vi "Ping_mean.vi"() -> ()   [LabVIEW 2018]
uses:
  <vilib>/Analysis/NI_AALBase.lvlib
panel:
  out "Distance (m)":dbl
  out "median":dbl format="%0.2f"
  in  "Count Integer":i32
  out "Last 10 (2)":dbl[](array[numeric]) format="%.3f"
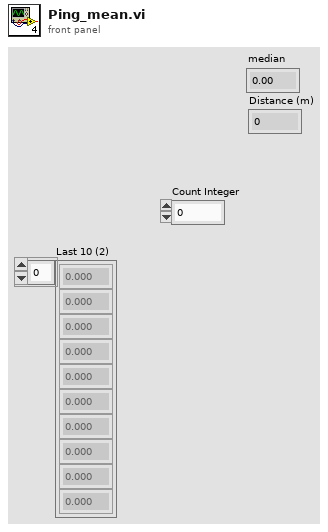
[diagram p1: front panel]
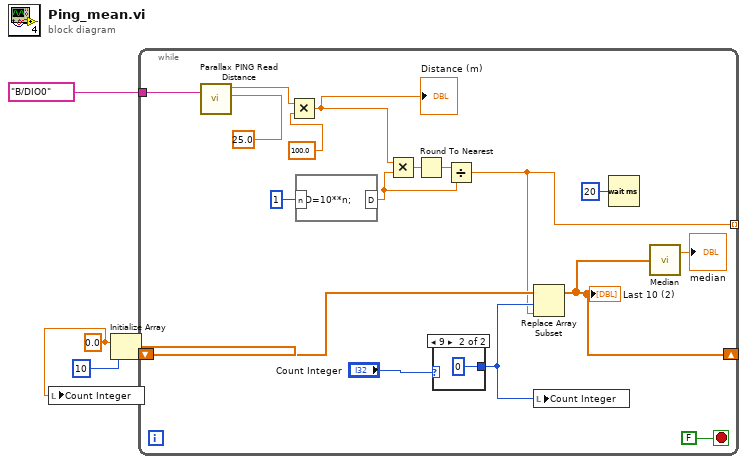
[diagram p0: block diagram]
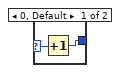
[diagram p2: hidden frame]
diagram:
  w2 = 0.0 ("element")
  n1 = local write "Count Integer"(w2) -> ()
  n2 = Initialize Array(w2, 10 ("dimension size")) -> (w3:dbl[])
  n3 = while {
    shift-right: [w16] -> _
    shift-left: w3 -> [w21]
    tunnel: [w10] -> _ mode=indexing
    tunnel: tag "B/DIO0" ("myRIO DIO Channel") -> [w5]
    stop <- FALSE stop-if-true
    n4 = call "Parallax PING Read Distance.vi"("Temperature (deg C)"=25.0, "myRIO DIO Channel"=w5) -> ("Distance (m)"=w7:dbl)  [unwired: 8 in, 1 out]
    n5 = Multiply(x=w7, y=100.0 ("Temperature (deg C)")) -> (x*y=w9:dbl)
    "Distance (m)" <- w9
    n6 = formula code="D=10**n;"("n"=u16 1 ("input variable")) -> ("D"=w12:dbl)
    n7 = Multiply(x=w9, y=w12) -> (x*y=w14:dbl)
    n8 = Round To Nearest(number=w14) -> (nearest integer value=w13:dbl)
    n9 = case shown="9" "Count Integer" {
      selector: "Count Integer" -> [w23 _]
      tunnel: [w22 0] -> w19
      frame 0, Default {
        n10 = Increment(x=w23) -> (x+1=w22:i32)
      }
      frame 9 {
      }
    }
    n11 = Divide(x=w13, y=w12) -> (x/y=w10:dbl)
    n12 = Replace Array Subset(array=w21, new element=w10, index=w19) -> (w16:dbl[])
    "Last 10 (2)" <- w16
    n13 = local write "Count Integer"(w19) -> ()
    n14 = Wait (ms)(milliseconds to wait=u32 20) -> ()  [unwired: 1 out]
    n15 = call <vilib>:"Median.vi"("X"=w16) -> ("median"=→"median":dbl)  [unwired: 1 out]
  }
